vi "ScriptSelectionDialog.vi"(8 "error in (no error)":errorcluster, 11 "WORef":T1) -> (0 "error out":errorcluster, 2 "Path":path, 3 "WORef Out":T1)   [LabVIEW 2011]
uses:
  Classes/WorkorderHandler/Software/DataStructures/WorkorderHandler_ObjectReference.ctl
  Strict Type Controls/Settings Operation.ctl
panel:
  in  "Script":string(combo)
  out "Quit":bool
  in  "OK":bool
  in  "OrderNo":string(combo)
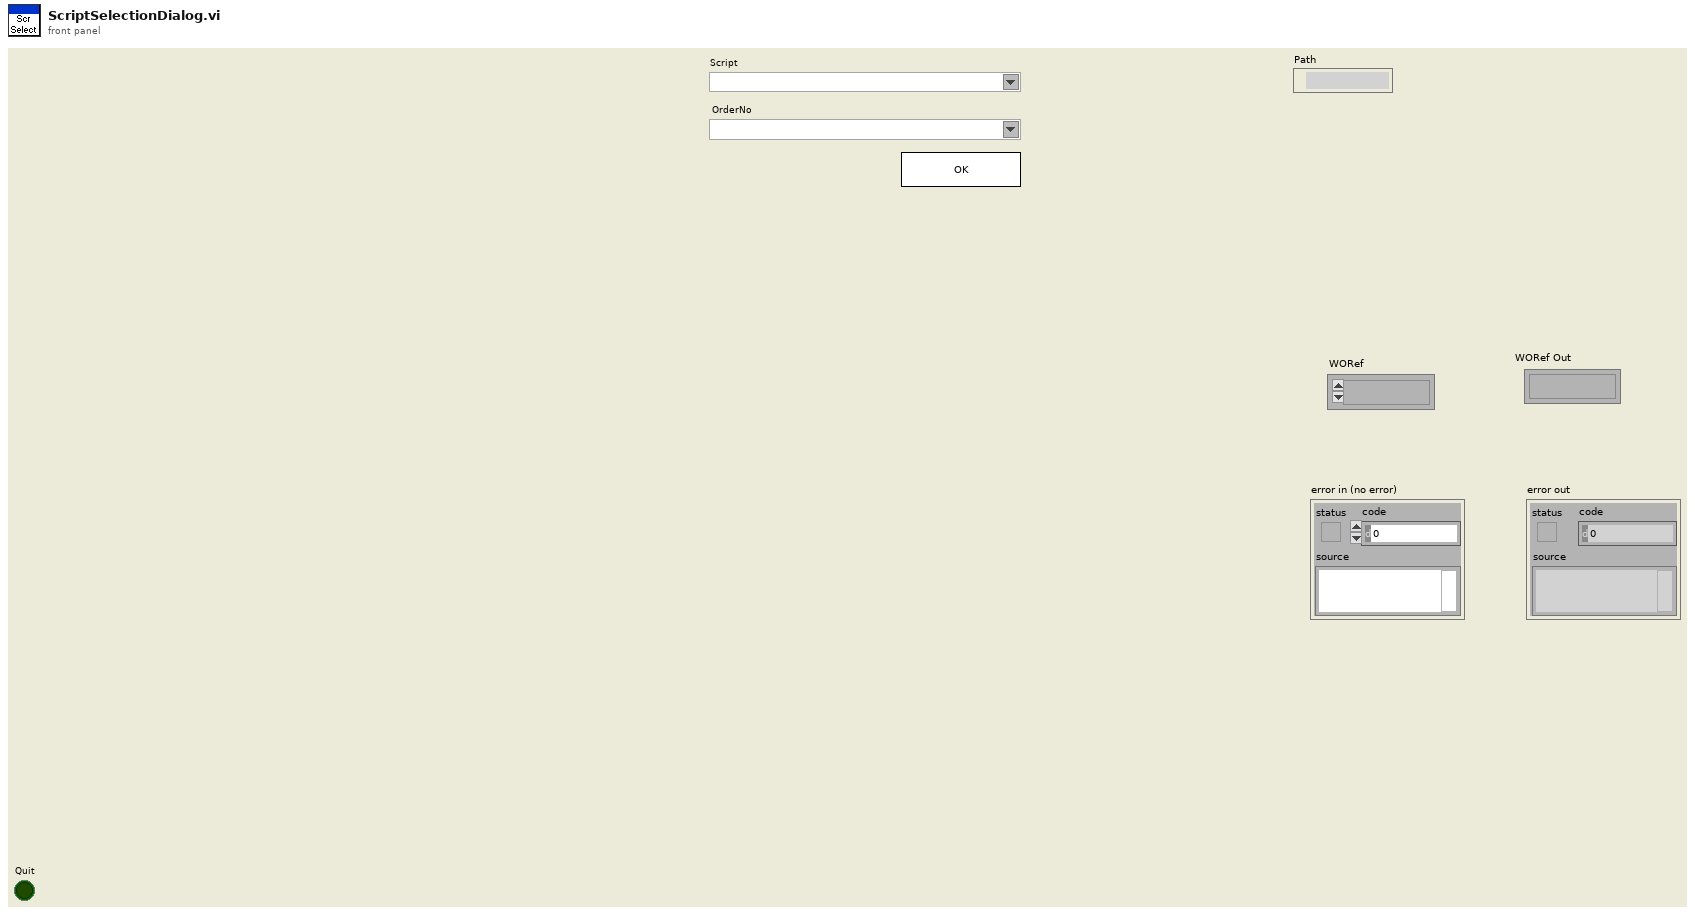
[diagram p1: front panel]
types:
  T1 = typedef "WorkorderHandler_ObjectReference.ctl" = refnum<k1>
  T2 = typedef "Settings Operation.ctl" = enum8{"Get Value", "Set Value", "Read File", "Write File", "Write Stored Value"}
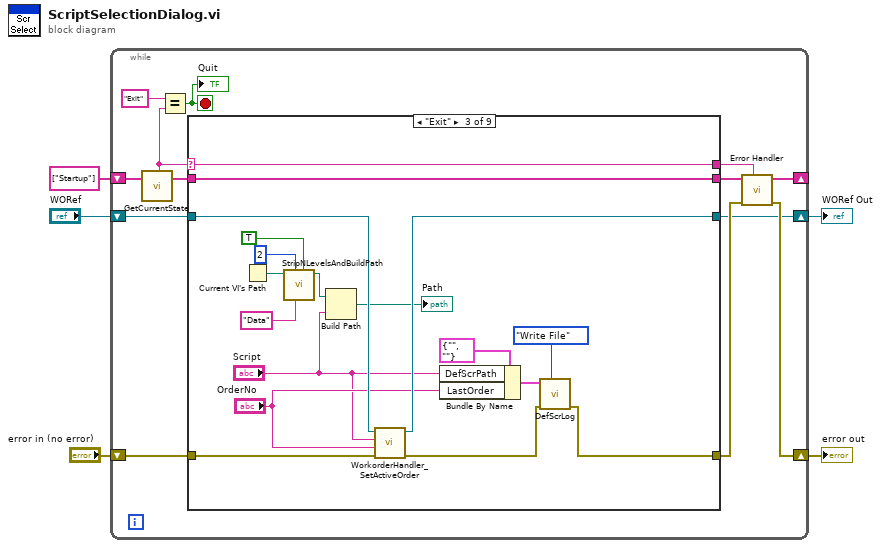
[diagram p0: block diagram]
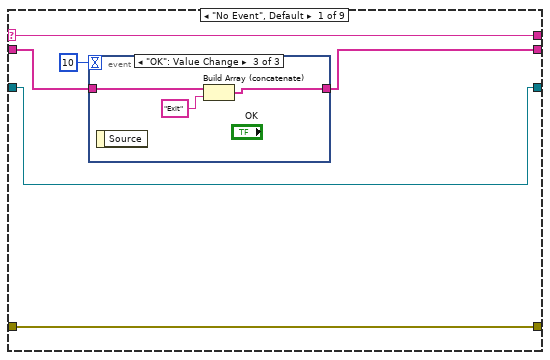
[diagram p2: hidden frame]
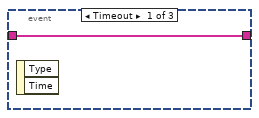
[diagram p3: hidden frame]
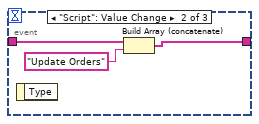
[diagram p4: hidden frame]
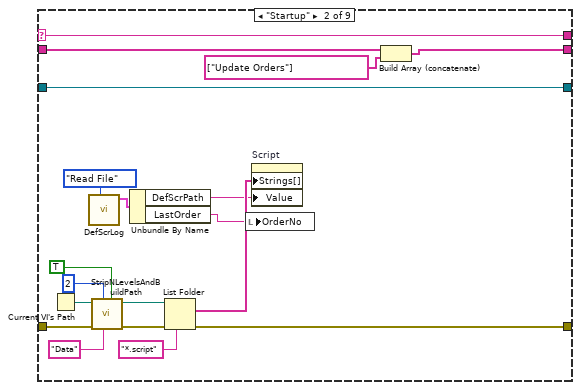
[diagram p5: hidden frame]
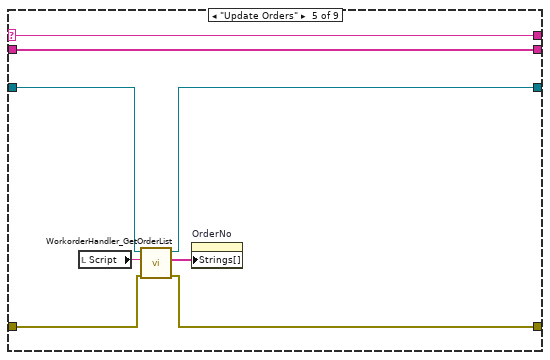
[diagram p7: hidden frame]
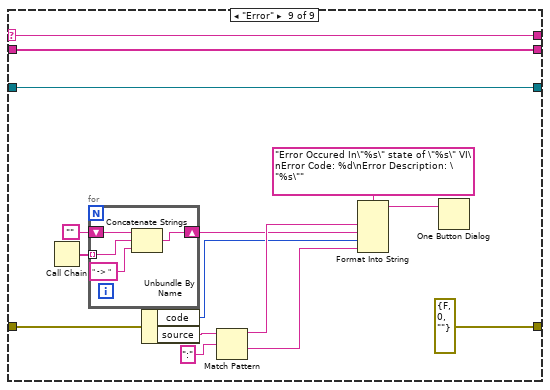
[diagram p11: hidden frame]
diagram:
  n1 = while {
    shift-right: [w14] -> _
    shift-left: string[] ["Startup"] ("State Array Out") -> [w18]
    shift-right: [w10] -> w3
    shift-left: "error in (no error)" -> [w11]
    shift-right: [w7] -> w1
    shift-left: "WORef" -> [w6]
    stop <- w15 stop-if-true
    n2 = call "GetCurrentState.vi"("State Array In"=w18) -> ("Current State"=w8:string, "State Array Out"=w17:string[])  [unwired: 1 in, 16 out]
    n3 = Equal?(x="Exit", y=w8) -> (x = y?=w15:bool)
    "Quit" <- w15
    n4 = case shown="\"Exit\"" w8 {
      selector: w8 -> [w24 w50 w68 w71 w79 w83 w87 w92 w107]
      tunnel: w17 -> [w23 w49 w67 w72 w80 w84 w88 w91 w94]
      tunnel: [w21 w48 w67 w72 w80 w84 w88 w91 w94] -> w13
      tunnel: [w20 w39 w60 w70 w75 w82 w86 w90 errorcluster {"status"=FALSE, "code"=0, "source"=""} ("error in (no error)")] -> w9
      tunnel: [w24 w50 w68 w71 w79 w83 w87 w92 w107] -> w12
      tunnel: w11 -> [w20 w42 w64 w70 w76 w82 w86 w90 w95]
      tunnel: [w19 w32 w65 w69 w77 w81 w85 w89 w93] -> w7
      tunnel: w6 -> [w19 w32 w66 w69 w78 w81 w85 w89 w93]
      frame "No Event", Default {
        n5 = event shown="[2] \"OK\": Value Change" {
          selector: _ -> [_ _ _]
          dyn-events: _ -> [_ _ _]
          timeout: 10 -> [_ _ _]
          tunnel: [w25 w27 w30] -> w21
          tunnel: w23 -> [w25 w28 w31]
          event Timeout {
            n6 = event-data() -> ()  [unwired: 3 out]
          }
          event "Script": Value Change {
            n7 = event-data() -> ()  [unwired: 2 out]
            n8 = Build Array (concatenate)(w28, "Update Orders" ("x")) -> (w27:string[])
          }
          event "OK": Value Change {
            n9 = event-data() -> ()  [unwired: 2 out]
            n10 = Build Array (concatenate)(w31, "Exit" ("x")) -> (w30:string[])
          }
        }
      }
      frame "Startup" {
        n11 = Current VI's Path() -> (path=w45:path)
        n12 = call "DefScrLog.vi"("Operation"=Settings_Operation."Read File") -> ("Def Settings Out"=w35:cluster{"DefScrPath":string, "LastOrder":string})  [unwired: 2 in, 8 out]
        n13 = call "StripNLevelsAndBuildPath.vi"("Create Folders"=TRUE, "Build Path"="Data" ("button label"), "Strip Levels"=2, "error in(no error)"=w42, "Path In"=w45) -> ("error out"=w40:errorcluster, "Path Out"=w41:path)  [unwired: 1 in, 4 out]
        n14 = Unbundle By Name(w35) -> ("DefScrPath"=w34:string, "LastOrder"=w33:string)
        n15 = List Folder(path=w41, pattern="*.script", error in=w40) -> (filenames=w37:string[], error out=w39:errorcluster)  [unwired: 3 out]
        n16 = local write "OrderNo"(w33) -> ()
        n17 = property on="Script" class="CmbBox"("Strings[]"=w37, "Value"=w34) -> ()  [unwired: 2 in, 2 out]
        n18 = Build Array (concatenate)(w49, string[] ["Update Orders"] ("State Array Out")) -> (w48:string[])
      }
      frame "Exit" {
        n19 = Current VI's Path() -> (path=w56:path)
        n20 = call "StripNLevelsAndBuildPath.vi"("Create Folders"=TRUE, "Build Path"="Data" ("button label"), "Strip Levels"=2, "Path In"=w56) -> ("Path Out"=w53:path)  [unwired: 2 in, 5 out]
        n21 = Build Path(base path=w53, name or relative path="Script") -> (appended path=→"Path":path)
        n22 = call "WorkorderHandler_SetActiveOrder.vi"("error in (no error)"=w64, "Order"="OrderNo", "Script"="Script", "reference"=w66) -> ("error out"=w61:errorcluster, "duplicate reference"=w65:T1)  [unwired: 6 out]
        n23 = Bundle By Name(cluster=cluster{"DefScrPath":string, "LastOrder":string} {"DefScrPath"="", "LastOrder"=""} ("input cluster"), "DefScrPath"="Script", "LastOrder"="OrderNo") -> (w62:cluster{"DefScrPath":string, "LastOrder":string})
        n24 = call "DefScrLog.vi"("Operation"=Settings_Operation."Write File", "error in (no error)"=w61, "Def Settings"=w62) -> ("error out"=w60:errorcluster)  [unwired: 8 out]
      }
      frame "---------------Below are UI Events---------------" {
        # "This State will never Execute\nIt is added just for improving code readability please do not remove this case"
      }
      frame "Update Orders" {
        n25 = local read "Script"() -> (w73:string)
        n26 = call "WorkorderHandler_GetOrderList.vi"("error in (no error)"=w76, "Script"=w73, "reference"=w78) -> ("error out"=w75:errorcluster, "Orders"=w74:string[], "duplicate reference"=w77:T1)  [unwired: 6 out]
        n27 = property on="OrderNo" class="CmbBox"("Strings[]"=w74) -> ()  [unwired: 2 in, 2 out]
      }
      frame "---------------Below are Menu Events---------------" {
        # "This State will never Execute\nIt is added just for improving code readability please do not remove this case"
      }
      frame "---------------Below are Subroutine states---------------" {
      }
      frame "---------------Below are Error Handling VIs---------------" {
      }
      frame "Error" {
        n28 = Call Chain() -> (call chain=w102:string[])
        n29 = for {
          tunnel: w102 -> [w110] mode=indexing
          shift-right: [w108] -> w99
          shift-left: "" -> [w111]
          n30 = Concatenate Strings(w111, w110, " -> ") -> (w108:string)
        }
        n31 = Unbundle By Name(w95) -> ("code"=w97:i32, "source"=w96:string)
        n32 = Match Pattern(string=w96, regular expression=":") -> (before substring=w100:string, after substring=w104:string)  [unwired: 3 out]
        n33 = Format Into String(format string="Error Occured In\"%s\" state of \"%s\" VI\nError Code: %d\nError Description: \"%s\"", w100, w99, w97, w104) -> (resulting string=w103:string)  [unwired: 2 in, 1 out]
        n34 = One Button Dialog(message=w103) -> ()  [unwired: 2 out]
      }
    }
    n35 = call "Error Handler.vi"("Current State"=w12, "error in (no error)"=w9, "Msg Queue In"=w13) -> ("error out"=w10:errorcluster, "Msg Queue Out"=w14:string[])  [unwired: 1 in, 6 out]
  }
  "error out" <- w3
  "WORef Out" <- w1
